vi "RT Strain Create Task.vi"(8 "error in":errorcluster, 11 "Data":T1={"AO config"=[], "AI config"=[], "DI config"=[], "DO config"=[], "TC config"=[], "ACC config"=[], "SG config"=[], "Strain Gauge Settings"={"poisson ratio"=0.3, "nominal gage resistance"=120.0, "gage factor"=2.08}, "Bridge Settings "={"strain configuration"=10271, "lead wire resistance"=1.7, "initial bridge voltage"=0.0, "voltage excitation source"=10200, "voltage excitation value"=3.3}, "Sample Rate"={"AI Sample Rate"=0.0, "AO Sample Rate"=0.0, "DI Sample Rate"=0.0, "TC Sample Rate"=0.0, "DO Sample Rate"=0.0, "SG Sample Rate"=0.0, "ACC Sample Rate"=0.0}} {"Bridge Settings"."strain configuration" items=["Full Bridge I"=10183, "Full Bridge II"=10184, "Full Bridge III"=10185, "Half Bridge I"=10188, "Half Bridge II"=10189, "Quarter Bridge I"=10271, "Quarter Bridge II"=10272]; "Bridge Settings"."voltage excitation source" items=["Internal"=10200, "External"=10167, "None"=10230]; "ACC config"."Terminal configuration" items=["default"=-1, "RSE"=10083, "NRSE"=10078, "Differential"=10106, "Pseudodifferential"=12529]; "ACC config"."Sensitivity units" items=["mVolts/g"=12509, "Volts/g"=12510]; "TC config"."type" items=["J"=10072, "K"=10073, "N"=10077, "R"=10082, "S"=10085, "T"=10086, "B"=10047, "E"=10055]; "TC config"."units" items=["Deg C", "Deg F", "Kelvins", "Deg R", "From Custom Scale"]}) -> (0 "error out":errorcluster, 2 "empty?":bool, 3 "task out":refnum<k21>)   [LabVIEW 2022 SP3]
uses:
  <vilib>/DAQmx/create/channels.llb/DAQmx Create Channel (AI-Strain-Strain Gage).vi
  RT Controls/RT Config.ctl
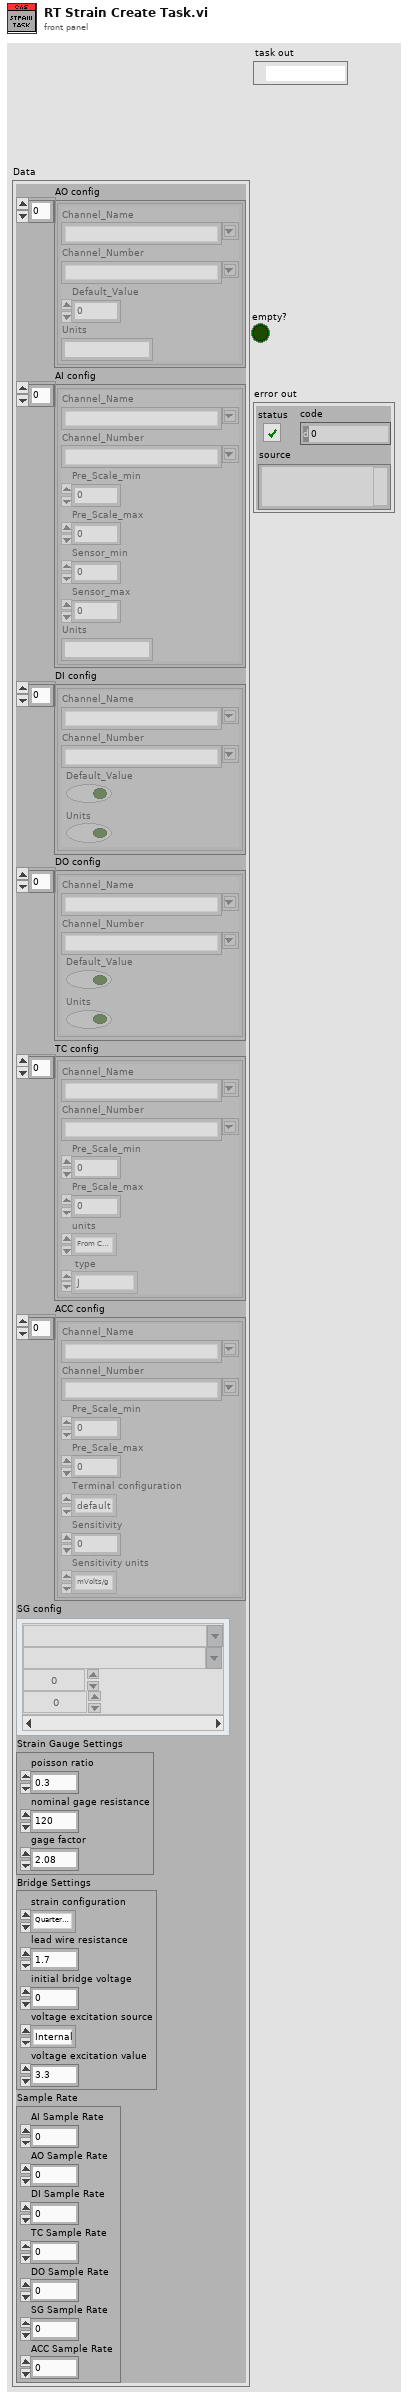
[diagram p1: front panel]
types:
  T1 = typedef "RT Config.ctl" = cluster{"AO config":cluster{"Channel_Name":string, "Channel_Number":string, "Default_Value":dbl, "Units":string}[], "AI config":cluster{"Channel_Name":string, "Channel_Number":string, "Pre_Scale_min":dbl, "Pre_Scale_max":dbl, "Sensor_min":dbl, "Sensor_max":dbl, "Units":string}[], "DI config":cluster{"Channel_Name":string, "Channel_Number":string, "Default_Value":bool, "Units":bool}[], "DO config":cluster{"Channel_Name":string, "Channel_Number":string, "Default_Value":bool, "Units":bool}[], "TC config":cluster{"Channel_Name":string, "Channel_Number":string, "Pre_Scale_min":dbl, "Pre_Scale_max":dbl, "units":i32, " type":i32}[], "ACC config":cluster{"Channel_Name":string, "Channel_Number":string, "Pre_Scale_min":dbl, "Pre_Scale_max":dbl, "Terminal configuration":i32, "Sensitivity":dbl, "Sensitivity units":i32}[], "SG config":cluster{"Channel_Name":string, "Channel_Number":string, "Pre_Scale_min":dbl, "Pre_Scale_max":dbl}[], "Strain Gauge Settings":cluster{"poisson ratio":dbl, "nominal gage resistance":dbl, "gage factor":dbl}, "Bridge Settings ":cluster{"strain configuration":i32, "lead wire resistance":dbl, "initial bridge voltage":dbl, "voltage excitation source":i32, "voltage excitation value":dbl}, "Sample Rate":cluster{"AI Sample Rate":dbl, "AO Sample Rate":dbl, "DI Sample Rate":dbl, "TC Sample Rate":dbl, "DO Sample Rate":dbl, "SG Sample Rate":dbl, "ACC Sample Rate":dbl}}
  T2 = cluster{"Channel_Name":string, "Channel_Number":string, "Pre_Scale_min":dbl, "Pre_Scale_max":dbl}[]
  T3 = cluster{"strain configuration":i32, "lead wire resistance":dbl, "initial bridge voltage":dbl, "voltage excitation source":i32, "voltage excitation value":dbl}
  T4 = cluster{"poisson ratio":dbl, "nominal gage resistance":dbl, "gage factor":dbl}
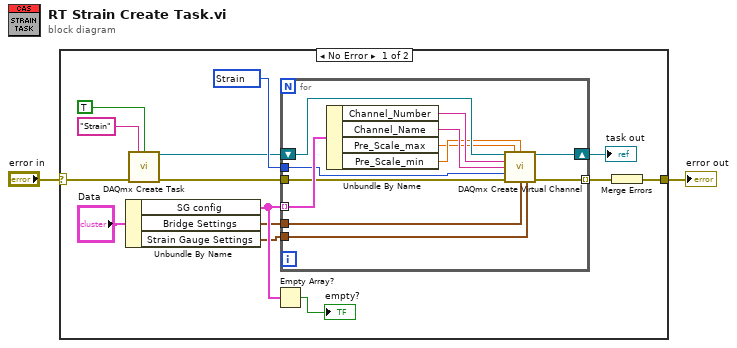
[diagram p0: block diagram]
diagram:
  n1 = case shown="No Error" "error in" {
    selector: "error in" -> [w13 w29]
    tunnel: [w9 w29] -> w1
    frame No Error {
      w16 = 10299 items=["Strain"=10299, "From Custom Scale"=10065] ("units")
      n2 = Unbundle By Name("Data") -> ("SG config"=w5:T2, "Bridge Settings"=w4:T3, "Strain Gauge Settings"=w3:T4)
      n3 = call <vilib>:"DAQmx Create Task.vi"("new task name"="Strain", "auto cleanup"=TRUE, "error in"=w13) -> ("task out"=w7:refnum<k21>, "error out"=w15:errorcluster)  [unwired: 11 in]
      n4 = Empty Array?(array=w5) -> (empty?=→"empty?":bool)
      n5 = for {
        shift-right: [w27] -> w10
        shift-left: w7 -> [w26]
        tunnel: w5 -> [w25] mode=indexing
        tunnel: w16 -> [w19]
        tunnel: w4 -> [w18]
        tunnel: w3 -> [w17]
        tunnel: w15 -> [w20]
        tunnel: [w28] -> w14 mode=indexing
        n6 = Unbundle By Name(w25) -> ("Channel_Number"=w24:string, "Channel_Name"=w23:string, "Pre_Scale_max"=w21:dbl, "Pre_Scale_min"=w22:dbl)
        n7 = call-poly <vilib>:"DAQmx Create Virtual Channel.vi"("task in"=w26, "maximum value"=w21, "minimum value"=w22, "physical channels"=w24, "name to assign"=w23, "units"=w19, "error in"=w20, "bridge information"=w18, "strain gage information"=w17) -> ("task out"=w27:refnum<k21>, "error out"=w28:errorcluster)  [unwired: 5 in]
      }
      "task out" <- w10
      n8 = Merge Errors(w14) -> (w9:errorcluster)
    }
    frame Error {
    }
  }
  "error out" <- w1
